vi "Final LCD Input (SubVI).vi"(8 "error in (no error)":errorcluster, 10 "String Input":string, 11 "state input":T1=enum."Shut") -> (0 "error out":errorcluster)   [LabVIEW 2017]
uses:
  controls/StatesEnum.ctl
  <vilib>/myRIO/Instrument Drivers/Onboard IO/UART/typedef/VISA Configuration.ctl
  <vilib>/Instr/_visa.llb/VISA Configure Serial Port (Instr).vi
  <vilib>/myRIO/Express VI/Onboard IO/UART/UART Express VI.xnode
  <vilib>/myRIO/Instrument Drivers/Onboard IO/UART/UART.lvlib
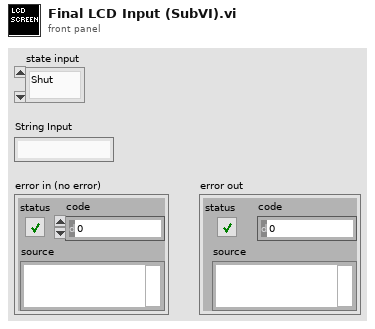
[diagram p1: front panel]
types:
  T1 = typedef "StatesEnum.ctl" = enum16{"Init", "Center Cliff\n", "Pause", "Drive", "L.Cliff", "R.Cliff", "Shut"}
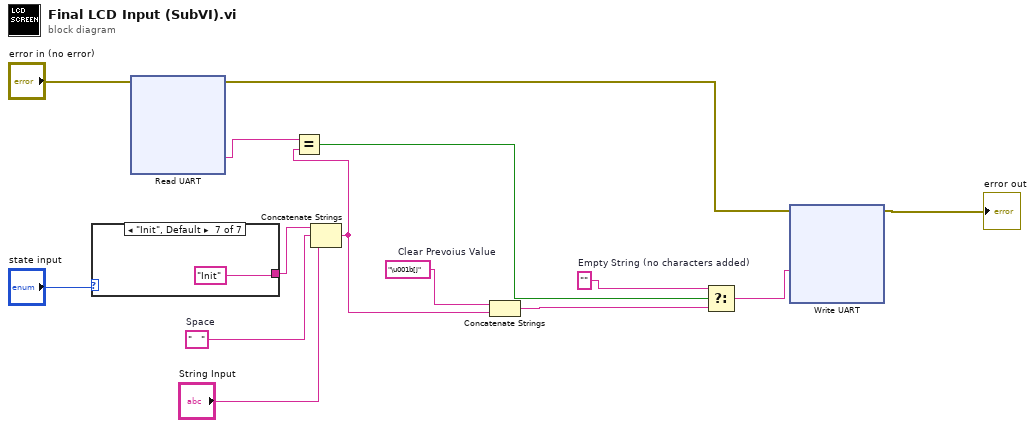
[diagram p0: block diagram]
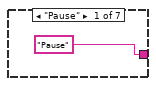
[diagram p2: hidden frame]
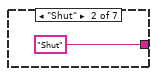
[diagram p3: hidden frame]
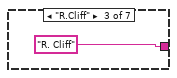
[diagram p4: hidden frame]
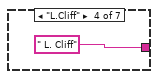
[diagram p5: hidden frame]
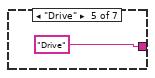
[diagram p6: hidden frame]
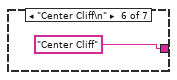
[diagram p7: hidden frame]
diagram:
  w13 = "   "  # Space
  w9 = "\u001b[j"  # Clear Prevoius Value
  w2 = ""  # Empty String (no characters added)
  n1 = case shown="\"Init\", Default" "state input" {
    tunnel: ["Pause" "Shut" "R. Cliff" " L. Cliff" "Drive" "Center Cliff" "Init"] -> w11
    frame "Pause" {
    }
    frame "Shut" {
    }
    frame "R.Cliff" {
    }
    frame "L.Cliff" {
    }
    frame "Drive" {
    }
    frame "Center Cliff\n" {
    }
    frame "Init", Default {
    }
  }
  n2 = xnode "Read UART"("error in (no error)"="error in (no error)") -> ("Characters Read"=w6:string, "error out"=w4:errorcluster)  [unwired: 1 in]
  n3 = Concatenate Strings(w11, w13, "String Input") -> (w14:string)
  n4 = Equal?(x=w6, y=w14) -> (x = y?=w3:bool)
  n5 = Concatenate Strings(w9, w14) -> (w10:string)
  n6 = Select(t=w2, s=w3, f=w10) -> (s? t:f=w1:string)
  n7 = xnode "Write UART"("Characters to Write"=w1, "error in (no error)"=w4) -> ("error out"=→"error out":errorcluster)  [unwired: 1 out]
